vi "PID FXP Template Single-Channel PID.vi"(0 "process variable":fxp<+/-,16,5>, 1 "reset?":bool, 7 "setpoint":fxp<+/-,16,5>, 12 "PID gains":T2={"proportional gain (Kc)"=127.99609375, "integral gain (Kc*Ts/Ti)"=127.99609375, "derivative gain (Kc*Td/Ts)"=0.0}, 13 "output range":T1={"output high"=15.99951171875, "output low"=-16.0}) -> (4 "output":fxp<+/-,16,16>)   [LabVIEW 2017]
doc: "On an FPGA target, implements an integer PID algorithm for PID applications with high-speed control and/or high channel count that require an efficient algorithm. You can use this Express VI with single-channel or multi-channel configurations. The PID algorithm features control action range and uses the integrator anti-windup calculation to limit the effect of the integral action during transients. The PID algorithm also features bumpless controller output for PID gain changes.\n--------------------------------------------------------\n\nThis Express VI is configured as follows:\n\nNumber of channels = 1\nProportional gain (Kc) = 1\nIntegral time (Ti) = 10mmin\nDerivative time (Td) = 0min\nSampling time (Ts) = 1s\nProportional gain (scaled) (Kc * 2^8) = 256\nIntegral gain (scaled) ([Kc*Ts]/[Ti*60] * 2^8) = 427\nDerivative gain (scaled) ([Kc*Td*60]/[Ts] * 2^8) = 0\nOutput range high = 32767\nOutput range low = -32768\nInitial setpoint = 0"
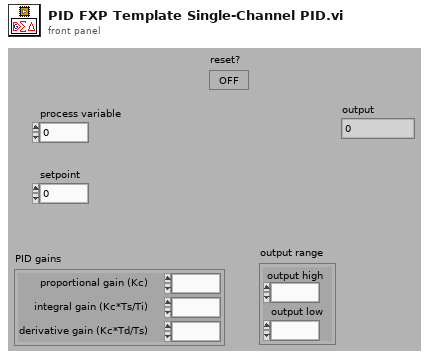
[diagram p1: front panel]
types:
  T1 = cluster{"output high":fxp<+/-,16,5>, "output low":fxp<+/-,16,5>}
  T2 = cluster{"proportional gain (Kc)":fxp<+/-,16,8>, "integral gain (Kc*Ts/Ti)":fxp<+/-,16,8>, "derivative gain (Kc*Td/Ts)":fxp<+/-,16,8>}
  T3 = cluster{"proportional gain (Kc)":i16, "integral gain (Kc*Ts/Ti)":i16, "derivative gain (Kc*Td/Ts)":i16}
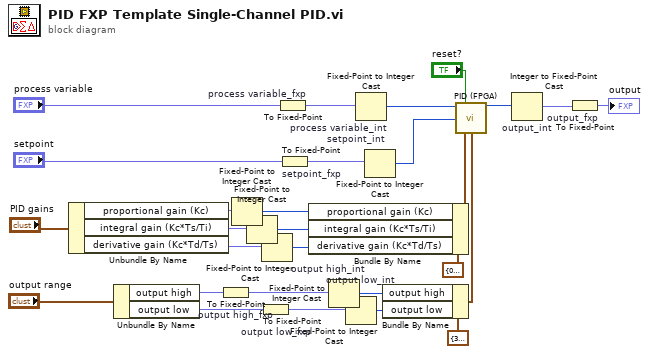
[diagram p0: block diagram]
diagram:
  n1 = Unbundle By Name("PID gains") -> ("proportional gain (Kc)"=w9:fxp<+/-,16,8>, "integral gain (Kc*Ts/Ti)"=w8:fxp<+/-,16,8>, "derivative gain (Kc*Td/Ts)"=w7:fxp<+/-,16,8>)
  n2 = Unbundle By Name("output range") -> ("output high"=w22:fxp<+/-,16,5>, "output low"=w23:fxp<+/-,16,5>)
  n3 = To Fixed-Point "output high_fxp"(number=w22) -> (fixed-point=w6:fxp<+/-,16,5>)  [unwired: 1 in]
  n4 = Fixed-Point to Integer Cast(1:w9) -> (0:w11:i16)
  n5 = Fixed-Point to Integer Cast(1:w8) -> (0:w10:i16)
  n6 = To Fixed-Point "output low_fxp"(number=w23) -> (fixed-point=w3:fxp<+/-,16,5>)  [unwired: 1 in]
  n7 = Fixed-Point to Integer Cast(1:w7) -> (0:w12:i16)
  n8 = To Fixed-Point "process variable_fxp"(number="process variable") -> (fixed-point=w15:fxp<+/-,16,5>)  [unwired: 1 in]
  n9 = To Fixed-Point "setpoint_fxp"(number="setpoint") -> (fixed-point=w14:fxp<+/-,16,5>)  [unwired: 1 in]
  n10 = Bundle By Name(cluster=T3 {"proportional gain (Kc)"=0, "integral gain (Kc*Ts/Ti)"=0, "derivative gain (Kc*Td/Ts)"=0} ("PID gains"), "proportional gain (Kc)"=w11, "integral gain (Kc*Ts/Ti)"=w10, "derivative gain (Kc*Td/Ts)"=w12) -> (w18:T3)
  n11 = Fixed-Point to Integer Cast "output high_int"(1:w6) -> (0:w5:i16)
  n12 = Fixed-Point to Integer Cast "output low_int"(1:w3) -> (0:w4:i16)
  n13 = Fixed-Point to Integer Cast "process variable_int"(1:w15) -> (0:w16:i16)
  n14 = Fixed-Point to Integer Cast "setpoint_int"(1:w14) -> (0:w13:i16)
  n15 = Bundle By Name(cluster=cluster{"output high":i16, "output low":i16} {"output high"=32767, "output low"=-32768} ("output range"), "output high"=w5, "output low"=w4) -> (w17:cluster{"output high":i16, "output low":i16})
  n16 = call "PID (FPGA).vi"("process variable"=w16, "reset?"="reset?", "setpoint"=w13, "PID gains"=w18, "output range"=w17) -> ("output"=w2:i16)  [unwired: 10 in]
  n17 = Integer to Fixed-Point Cast "output_int"(integer=w2) -> (fixed-point=w1:fxp<+/-,16,16>)  [unwired: 1 in]
  n18 = To Fixed-Point "output_fxp"(number=w1) -> (fixed-point=→"output":fxp<+/-,16,16>)  [unwired: 1 in]
